vi "MOVE BIAS.vi"(0 "ScanQ in":refnum<queue>, 1 "return value":cluster{"x":dbl, "y":dbl}, 5 "Initial X":sgl, 7 "Boolean":bool, 9 "Initial Y":sgl, 11 "error in (no error)":errorcluster) -> (4 "ScanQ out":refnum<queue>, 6 "FInal X (m)":sgl, 10 "Final Y (m)":sgl, 15 "error out":errorcluster)   [LabVIEW 2025]
uses:
  CTL's/Scan_Params (QMH).ctl
  Bias Cont QMH.ctl
panel:
  out "Bias out 2":T1 {"Final Y (m)" format="%.3p"; "Final X (m)" format="%.3p"}
  in  "Bias in":T1 {"Final Y (m)" format="%.3p"; "Final X (m)" format="%.3p"}
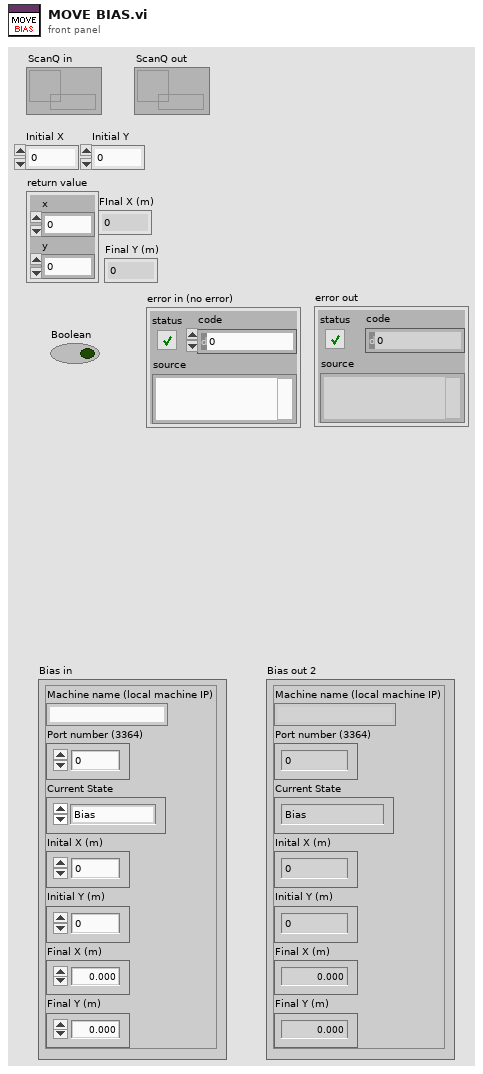
[diagram p1: front panel]
types:
  T1 = typedef "Bias Cont QMH.ctl" = cluster{"Machine name (local machine IP)":string, "Port number (3364)":u32, "Current State":enum16{"Bias", "Stop"}, "Inital X (m)":dbl, "Initial Y (m)":dbl, "Final X (m)":sgl, "Final Y (m)":sgl}
  T2 = enum16{"1. BIAS", "2. INIT_SCAN", "3. SCAN_IDLE", "4. INTER_SCAN", "5. NEW_COORDS_&_FRAME", "6. FINAL_SCAN", "7. POLL_BIAS", "8. Z-CONT.", "9. STOP"}
  T3 = typedef "Scan_Params (QMH).ctl" = cluster{"Setpoint (I)":dbl[], "Bias (V)":dbl[], "Number of scans":u8, "Port number (3364)":u32, "Avoid zero threshold (V)":dbl, "Current State":enum16{"1. BIAS", "2. INIT_SCAN", "3. SCAN_IDLE", "4. INTER_SCAN", "5. NEW_COORDS_&_FRAME", "6. FINAL_SCAN", "7. POLL_BIAS", "8. Z-CONT.", "9. STOP"}}
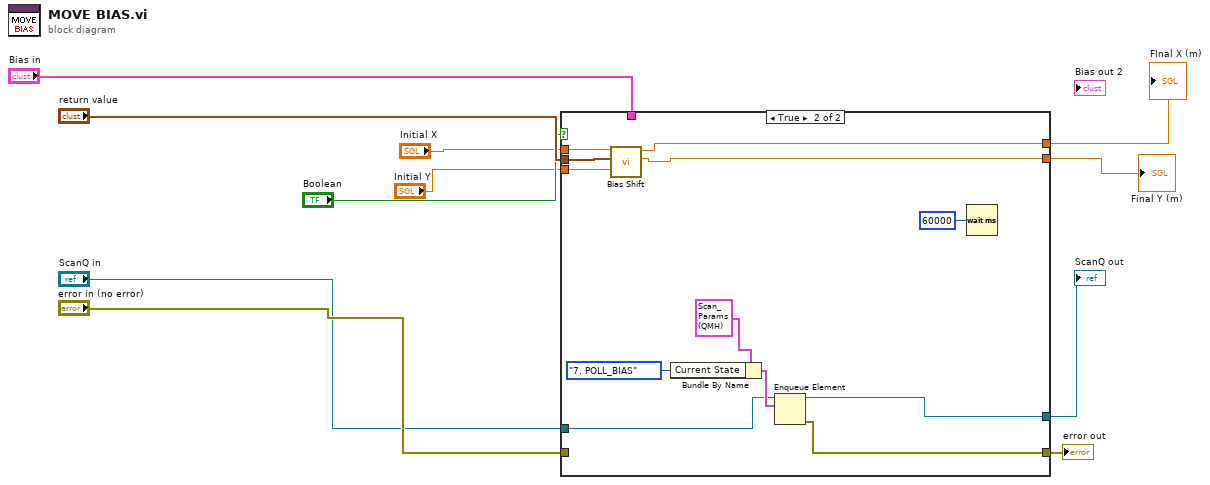
[diagram p0: block diagram]
diagram:
  n1 = case shown="True" "Boolean" {
    tunnel: "return value" -> [_ w24]
    tunnel: "ScanQ in" -> [w13 w17]
    tunnel: [w13 w15] -> w9
    tunnel: [w12 w16] -> w1
    tunnel: "error in (no error)" -> [w12 _]
    tunnel: [_ w23] -> w2
    tunnel: "Bias in" -> [_ _]
    tunnel: "Initial X" -> [_ w22]
    tunnel: "Initial Y" -> [_ w21]
    tunnel: [_ w20] -> w3
    frame False {
    }
    frame True {
      n2 = call "Bias Shift.vi"("Initial Y"=w21, "Translation (m)"=w24, "Initial X"=w22) -> ("Final Y (m)"=w20:sgl, "FInal X (m)"=w23:sgl)  [unwired: 7 in]
      n3 = Bundle By Name(cluster=T3 {"Setpoint (I)"=[], "Bias (V)"=[], "Number of scans"=1, "Port number (3364)"=3364, "Avoid zero threshold (V)"=0.004999999888241291, "Current State"=enum."1. BIAS"} ("element"), "Current State"=T2."7. POLL_BIAS") -> (w18:T3)
      n4 = Enqueue Element(queue=w17, element=w18) -> (queue out=w15:refnum<queue>, error out=w16:errorcluster)  [unwired: 2 in, 1 out]
      n5 = Wait (ms)(milliseconds to wait=u32 60000) -> ()  [unwired: 1 out]
    }
  }
  "ScanQ out" <- w9
  "Final Y (m)" <- w3
  "FInal X (m)" <- w2
  "error out" <- w1
